vi "Set Horizontal Scale.vi"(8 "error in (no error)":errorcluster, 10 "Secs/div":dbl, 11 "VISA resource name":refnum<visa-resource-name>) -> (0 "error out":errorcluster, 3 "VISA resource name out":refnum<visa-resource-name>)   [LabVIEW 2018, in "DPO4104.lvlib" / "DPO4104.lvclass"]
doc: "This VI sends the command to set the seconds per division."
uses:
  DPO4104.lvclass
  <instrlib>/Tektronix DPO MSO 2000 4000 Series/Tektronix DPO MSO 2000 4000 Series.lvlib
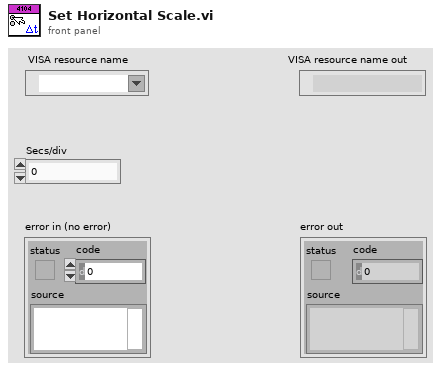
[diagram p1: front panel]
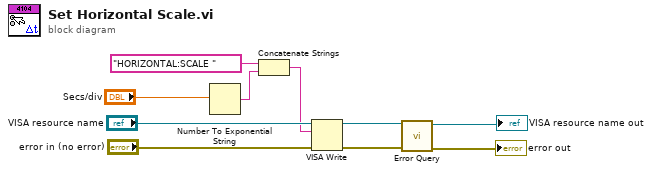
[diagram p0: block diagram]
diagram:
  n1 = Number To Exponential String(number="Secs/div") -> (E-format string=w6:string)  [unwired: 3 in]
  n2 = Concatenate Strings("HORIZONTAL:SCALE ", w6) -> (w3:string)
  n3 = VISA Write(VISA resource name="VISA resource name", write buffer=w3, error in (no error)="error in (no error)") -> (VISA resource name out=w2:refnum<visa-resource-name>, error out=w1:errorcluster)  [unwired: 1 out]
  n4 = call <instrlib>:"Error Query.vi"("error in (no error)"=w1, "VISA resource name"=w2) -> ("error out"=→"error out":errorcluster, "VISA resource name out"=→"VISA resource name out":refnum<visa-resource-name>)  [unwired: 6 in, 2 out]
